vi "Periodic Tasks.vi"() -> ()   [LabVIEW 2016]
doc: "This VI runs in parallel to other tasks. It can contain as many user-defined periodic loops as you need. These can carry out PID or other sorts of timed response."
uses:
  Refname/Swerve Motors.ctl
  Refname/Drive Motors.ctl
  Refname/Refname to String (Swerve).vi
  Refname/Refname to String (Drive).vi
  Robot Global Data.vi
panel:
  out "error out":errorcluster
  in  "error in":errorcluster
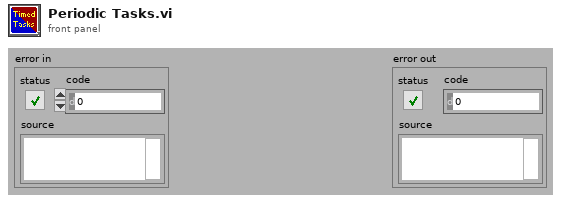
[diagram p1: front panel]
types:
  T1 = typedef "Drive Motors.ctl" = enum16{"Drive 1", "Drive 2", "Drive 3", "Drive 4"}
  T2 = typedef "Swerve Motors.ctl" = enum16{"Swerve 1", "Swerve 2", "Swerve 3", "Swerve 4"}
  T3 = typedef "WPI_MotorControlDeviceRef.ctl" = cluster{"DeviceStatus":errorcluster, "Type":T4, "PWM":cluster{"PWM Channel":T5, "DeadBand":T6}, "CAN":cluster{"Device Number":u8, "SetOutput VI Ref":variant, "GetOutput VI Ref":variant, "Enable VI Ref":variant, "Disable VI Ref":variant, "Data":variant}, "Invert":bool}
  T4 = typedef "WPI_MotorControlType.ctl" = enum16{"PWM", "CAN"}
  T5 = typedef "FPGA_DIOPWMChannel.ctl" = enum8{"PWM 0", "PWM 1", "PWM 2", "PWM 3", "PWM 4", "PWM 5", "PWM 6", "PWM 7", "PWM 8", "PWM 9", "PWM MXP 0", "PWM MXP 1", "PWM MXP 2", "PWM MXP 3", "PWM MXP 4", "PWM MXP 5", "PWM MXP 6", "PWM MXP 7", "PWM MXP 8", "PWM MXP 9", "Invalid"}
  T6 = typedef "WPI_PWMDeadband.ctl" = cluster{"Name":string, "maxPositivePwm":i32, "minPositivePwm":i32, "centerPwm":i32, "maxNegativePwm":i32, "minNegativePwm":i32, "angularRange":u16}
  T7 = cluster{"X":dbl, "Y":dbl, "Z":dbl, "Straight Drive":bool, "Reverse Drive":bool, "Low Sensitivity":bool, "Button A":bool, "Button B":bool}
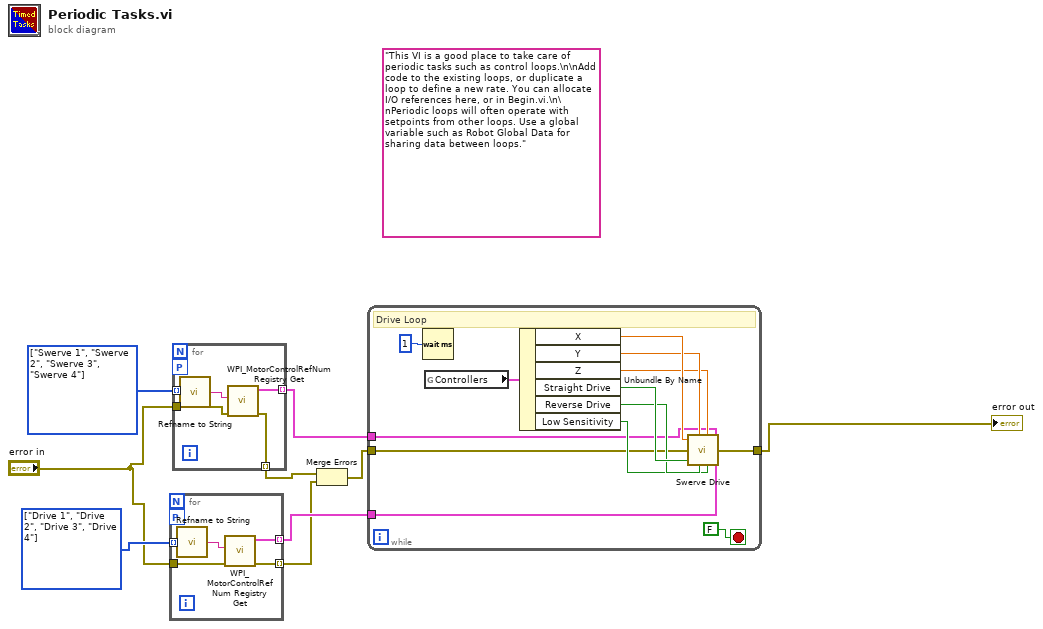
[diagram p0: block diagram]
diagram:
  w9 = T1[] [enum."Drive 1", enum."Drive 2", enum."Drive 3", enum."Drive 4"] items=["Drive 1", "Drive 2", "Drive 3", "Drive 4"]
  w8 = T2[] [enum."Swerve 1", enum."Swerve 2", enum."Swerve 3", enum."Swerve 4"] items=["Swerve 1", "Swerve 2", "Swerve 3", "Swerve 4"]
  (unwired) "This VI is a good place to take care of periodic tasks such as control loops.\n\nAdd code to the existing loops, or duplicate a loop to define a new rate. You can allocate I/O references here, or in Begin.vi.\n\nPeriodic loops will often operate with setpoints from other loops. Use a global variable such as Robot Global Data for sharing data between loops."
  n1 = for {
    workers-P: _ -> [_]
    tunnel: [w13] -> w7 mode=indexing
    tunnel: w9 -> [w12] mode=indexing
    tunnel: "error in" -> [w11]
    tunnel: [w10] -> w3 mode=indexing
    n2 = call-poly "Refname to String.vi"("Enum"=w12) -> ("resulting string"=w14:string)
    n3 = call <vilib>:"WPI_MotorControlRefNum Registry Get.vi"("error in (no error)"=w11, "refnum name"=w14) -> ("error out"=w10:errorcluster, "MotorControlDevRef"=w13:T3)  [unwired: 8 in]
  }
  n4 = for {
    workers-P: _ -> [_]
    tunnel: [w18] -> w6 mode=indexing
    tunnel: w8 -> [w17] mode=indexing
    tunnel: "error in" -> [w16]
    tunnel: [w15] -> w4 mode=indexing
    n5 = call-poly "Refname to String.vi"("Enum"=w17) -> ("String"=w19:string)
    n6 = call <vilib>:"WPI_MotorControlRefNum Registry Get.vi"("error in (no error)"=w16, "refnum name"=w19) -> ("error out"=w15:errorcluster, "MotorControlDevRef"=w18:T3)  [unwired: 8 in]
  }
  n7 = Merge Errors(w4, w3) -> (w2:errorcluster)
  n8 = while {
    tunnel: w7 -> [w25]
    tunnel: w6 -> [w24]
    tunnel: w2 -> [w21]
    tunnel: [w20] -> w1
    stop <- FALSE stop-if-true
    # "Drive Loop"
    n9 = Wait (ms)(milliseconds to wait=u32 1) -> ()  [unwired: 1 out]
    n10 = global read "Robot Global Data.vi" "Controllers"() -> (w32:T7)
    n11 = Unbundle By Name(w32) -> ("X"=w31:dbl, "Y"=w30:dbl, "Z"=w29:dbl, "Straight Drive"=w28:bool, "Reverse Drive"=w27:bool, "Low Sensitivity"=w26:bool)
    n12 = call "Swerve Drive.vi"("X"=w31, "Y"=w30, "error in"=w21, "Straight Drive"=w28, "Reverse Drive"=w27, "Z"=w29, "Swerve Dev Ref"=w24, "Low Sensitivity"=w26, "Drive Dev Ref"=w25) -> ("error out"=w20:errorcluster)
  }
  "error out" <- w1
